vi "SpecAnMeasCW_Cal.vi"(0 "VISA Refnum in":refnum<visa-resource-name>="GPIB0::18::INSTR", 1 "IsPSA(t)":bool, 2 "Use PK Search (T)":bool, 5 "SET CF (MHz) in":dbl, 11 "error in (no error)":errorcluster {"code" format="%.0x"}) -> (4 "VISA Refnum out":refnum<visa-resource-name>, 8 "Freq":dbl, 10 "Ampl":dbl, 14 "Mark Values":dbl[](array[numeric]), 15 "error out":errorcluster {"code" format="%.0x"})   [LabVIEW 2018]
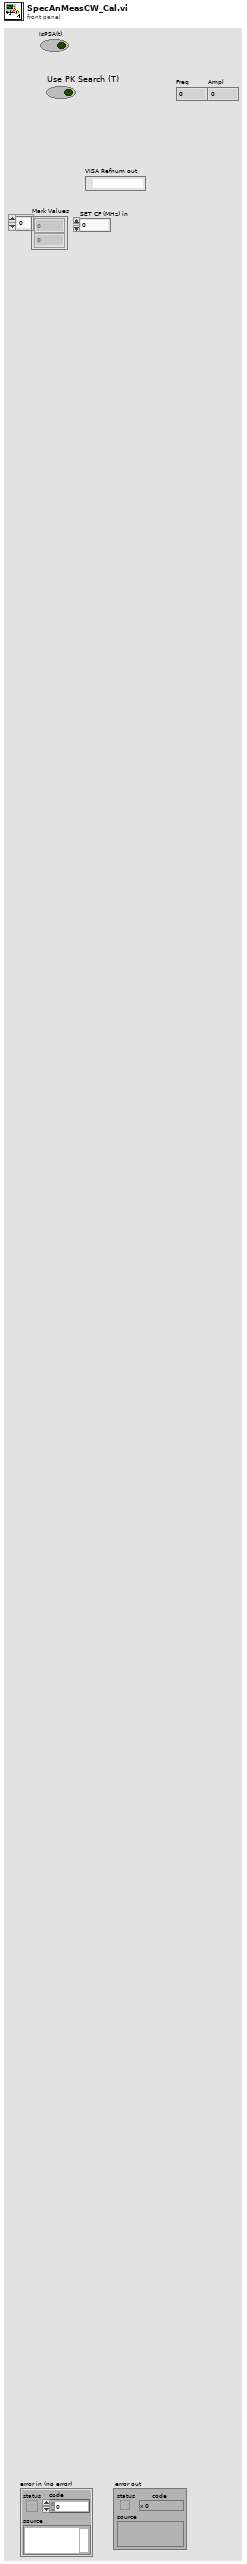
[diagram p1: front panel]
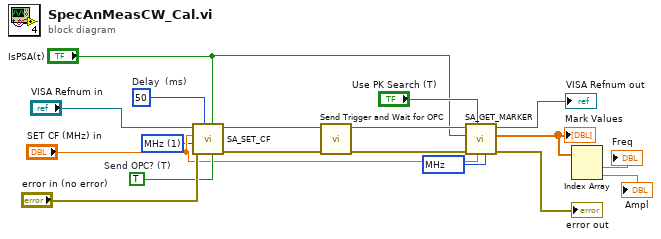
[diagram p0: block diagram]
diagram:
  w1 = u16 1 items=["Hz", "MHz", "GHz"] ("Freq Units")
  w2 = i64 1000000 items=["Hz"=1, "KHz"=1000, "MHz"=1000000, "GHz"=1000000000] ("Units")
  w6 = TRUE  # Send OPC? (T)
  w7 = i64 50  # Delay  (ms)
  n1 = call "SA_SET_CF.vi"("Send OPC? (T)"=w6, "IsPSA(t)"="IsPSA(t)", "Delay  (ms)"=w7, "error in"="error in (no error)", "Freq Units"=w1, "SET CF ()"="SET CF (MHz) in", "Session In"="VISA Refnum in") -> ("error out"=w13:errorcluster, "Session Out"=w12:refnum<visa-resource-name>)  [unwired: 2 in, 1 out]
  n2 = call "Send Trigger and Wait for OPC.vi"("error in"=w13, "Session In"=w12) -> ("error out"=w14:errorcluster, "Session Out"=w11:refnum<visa-resource-name>)  [unwired: 7 in, 1 out]
  n3 = call "SA_GET_MARKER.vi"("Units"=w2, "Set MKR Freq ()"="SET CF (MHz) in", "Use PK Search (T)"="Use PK Search (T)", "error in"=w14, "IsPSA?(t)"="IsPSA(t)", "Session In"=w11) -> ("error out"=→"error out":errorcluster, "Mark Values"=w10:dbl[], "Session Out"=→"VISA Refnum out":refnum<visa-resource-name>)  [unwired: 2 in, 1 out]
  "Mark Values" <- w10
  n4 = Index Array(array=w10) -> (element #1=→"Freq":dbl, element #2=→"Ampl":dbl)  [unwired: 2 in]
